vi "FrameRef to Sigs.vi"(8 "error in (no error)":errorcluster, 11 "Data in":T1[](array[typedef])) -> (0 "error out":errorcluster, 3 "Signals":T1[](array[typedef]))   [LabVIEW 2021]
uses:
  <resource>/objmgr/xnet.rc
  <vilib>/xnet/xnet.llb/XNET Frame Type CAN.ctl
  <vilib>/xnet/xnet.llb/XNET Frame CAN.ctl
  controls/Signal Data.ctl
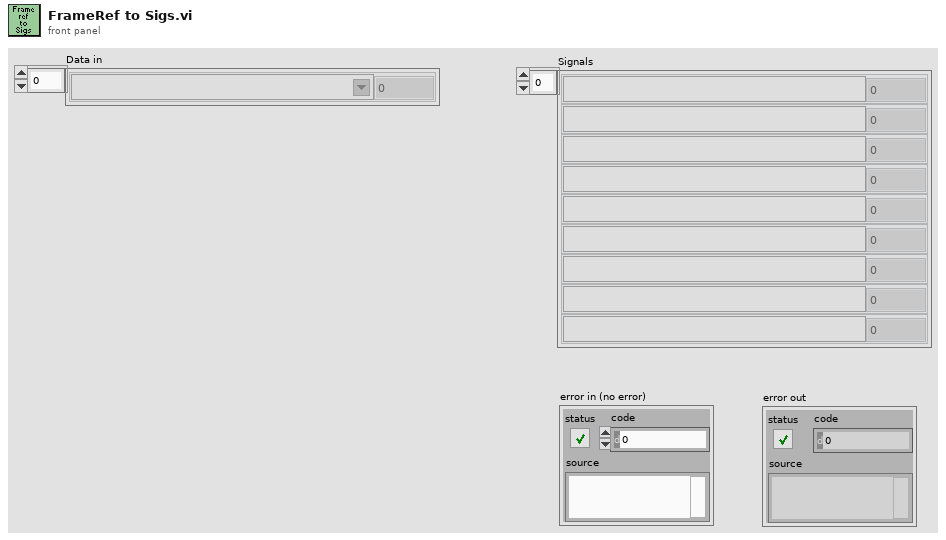
[diagram p1: front panel]
types:
  T1 = typedef "Signal Data.ctl" = cluster{"XNET Signal":refnum<k21>, "Data":dbl}
  T2 = typedef "XNET Frame CAN.ctl" = cluster{"timestamp":timestamp, "payload":u8[], "identifier":u32, "type":T3, "extended?":bool, "echo?":bool}
  T3 = typedef "XNET Frame Type CAN.ctl" = u8
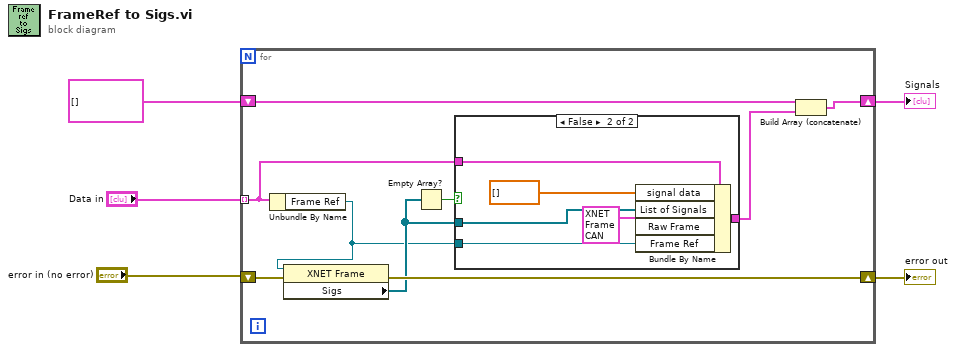
[diagram p0: block diagram]
diagram:
  n1 = for {
    shift-right: [w13] -> w4
    shift-left: T1[] [] ("Array") -> [w14]
    shift-right: [w12] -> w3
    shift-left: "error in (no error)" -> [w10]
    tunnel: "Data in" -> [w7] mode=indexing
    n2 = Unbundle By Name(w7) -> ("Frame Ref"=w6:refnum<k21>)
    n3 = property class="XNET Frame"(reference=w6, error in=w10) -> (error out=w12:errorcluster, "Sigs"=w8:refnum<k21>[])  [unwired: 1 out]
    n4 = Empty Array?(array=w8) -> (empty?=w9:bool)
    n5 = case shown="False" w9 {
      tunnel: [w15 w21] -> w11
      tunnel: w8 -> [_ w19]
      tunnel: w7 -> [w15 w17]
      tunnel: w6 -> [_ w16]
      frame True {
        # "some frames have\nno signals\nwill cause an \nerror when starting\nconversion"
      }
      frame False {
        n6 = Bundle By Name(cluster=w17, "signal data"=dbl[] [], "List of Signals"=w19, "Raw Frame"=T2 {"timestamp"=timestamp(0 s since 1904-01-01), "payload"=[], "identifier"=0, "type"=0, "extended?"=FALSE, "echo?"=FALSE} ("CAN frame"), "Frame Ref"=w16) -> (w21:T1)
      }
    }
    n7 = Build Array (concatenate)(w14, w11) -> (w13:T1[])
  }
  "Signals" <- w4
  "error out" <- w3
